vi "FTW-Time-Remaining.vi"(0 "Total Work Units":i64, 5 "Work Units Complete":i64, 7 "Initial Timer Value":dbl format="%.4psec", 11 "Window Size (for smoothing)":i32=15) -> (4 "Fraction Done [0.0,1.0]":dbl, 6 "Elapsed Time":dbl format="%.4psec", 8 "Estimated Time Remaining":dbl format="%.4psec", 10 "Current Rate (work/sec)":dbl, 15 "Settled?":bool)   [LabVIEW 2015]
panel:
  # "Inputs"
  # "Outputs"
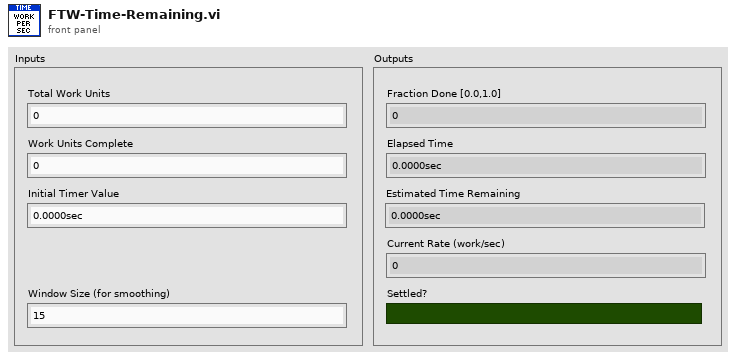
[diagram p1: front panel]
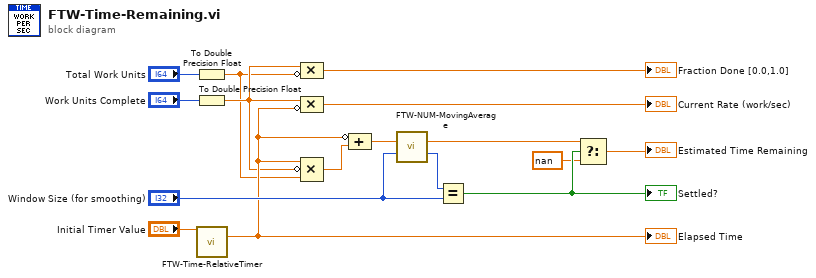
[diagram p0: block diagram]
diagram:
  n1 = To Double Precision Float(number="Total Work Units") -> (double precision float=w1:dbl)
  n2 = To Double Precision Float(number="Work Units Complete") -> (double precision float=w2:dbl)
  n3 = call "FTW-Time-RelativeTimer.vi"("Previous Timer Value"="Initial Timer Value") -> ("Elapsed Time"=w4:dbl)  [unwired: 12 in, 2 out]
  "Elapsed Time" <- w4
  n4 = Compound Arithmetic op=MULTIPLY(w2, invert w1) -> (→"Fraction Done [0.0,1.0]":dbl)
  n5 = Compound Arithmetic op=MULTIPLY(w2, invert w4) -> (→"Current Rate (work/sec)":dbl)
  n6 = Compound Arithmetic op=MULTIPLY(w4, invert w2, w1) -> (w16:dbl)
  n7 = Compound Arithmetic op=ADD(invert w4, w16) -> (w11:dbl)
  n8 = call "FTW-NUM-MovingAverage.vi"("New Value"=w11, "Window Size"="Window Size (for smoothing)") -> ("Average Value"=w6:dbl, "Items in Window"=w10:i32)  [unwired: 11 in, 1 out]
  n9 = Equal?(x=w10, y="Window Size (for smoothing)") -> (x = y?=w8:bool)
  "Settled?" <- w8
  n10 = Select(t=w6, s=w8, f=nan) -> (s? t:f=→"Estimated Time Remaining":dbl)
